vi "Equipe.vi"() -> (0 "port":i32, 1 "DA":string, 2 "设备名":string, 3 "AD":string)   [LabVIEW 2018]
panel:
  out "子字符串之前":string
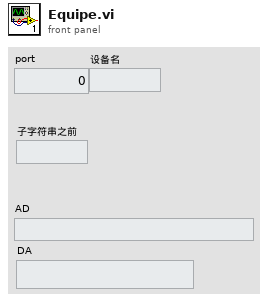
[diagram p1: front panel]
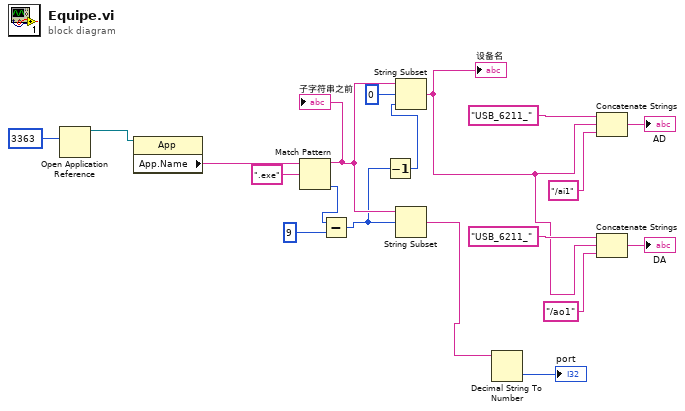
[diagram p0: block diagram]
diagram:
  n1 = Open Application Reference(10:u16 3363 ("端口号或服务名称(3363)")) -> (3:w19:refnum<vi>)  [unwired: 3 in, 1 out]
  n2 = property class="App"(reference=w19) -> ("App.Name"=w17:string)  [unwired: 1 in, 2 out]
  n3 = Match Pattern(string=w17, regular expression=".exe" ("正则表达式")) -> (before substring=w7:string, offset past match=w9:i32)  [unwired: 1 in, 2 out]
  "子字符串之前" <- w7
  n4 = Subtract(x=w9, y=9) -> (x-y=w4:i32)
  n5 = Decrement(x=w4) -> (x-1=w3:i32)
  n6 = String Subset(string=w7, offset (0)=0 ("偏移量(0)"), length (rest)=w3) -> (substring=w5:string)
  "设备名" <- w5
  n7 = String Subset(string=w7, offset (0)=w4) -> (substring=w2:string)  [unwired: 1 in]
  n8 = Decimal String To Number(string=w2) -> (number=→"port":i32)  [unwired: 2 in, 1 out]
  n9 = Concatenate Strings("USB_6211_", w5, "/ai1" ("字符串")) -> (→"AD":string)
  n10 = Concatenate Strings("USB_6211_", w5, "/ao1" ("字符串")) -> (→"DA":string)
